vi "tcp_prepare_mode.vi"(0 "button_tcp_vna_mode":bool, 5 "button_tcp_s11_mode":bool, 7 "button_tcp_s21_mode":bool, 9 "button_tcp_smith_mode":bool, 12 "sweep_start":dbl, 13 "sweep_stop":dbl, 14 "sweep_points":dbl) -> (4 "mode":string, 6 "data_out":T1)   [LabVIEW 2025]
uses:
  2542fa05-10a6-4b30-b761-6670dfe4c8c8.vi
  647f14ae-cfaa-4bfc-9393-0c1ebd99a498.vi
  f7317db9-9ae3-40bd-acdc-ae7c641fa7e1.vi
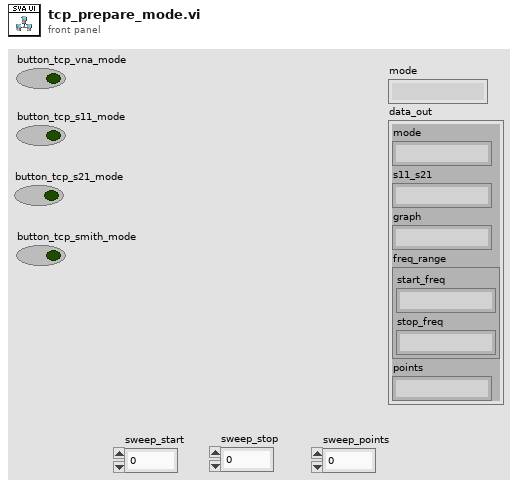
[diagram p1: front panel]
types:
  T1 = cluster{"mode":string, "s11_s21":string, "graph":string, "freq_range":cluster{"start_freq":string, "stop_freq":string}, "points":string}
  T2 = cluster{string, string, string, cluster{string, string}, string}
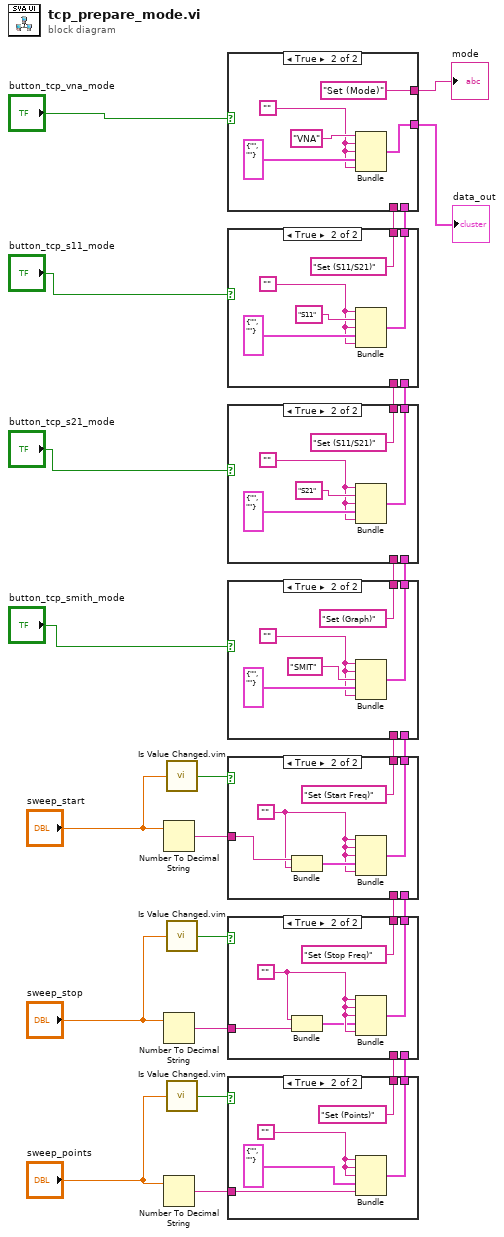
[diagram p0: block diagram]
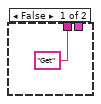
[diagram p2: hidden frame]
diagram:
  n1 = Number To Decimal String(number="sweep_start") -> (decimal integer string=w19:string)  [unwired: 1 in]
  n2 = Number To Decimal String(number="sweep_stop") -> (decimal integer string=w25:string)  [unwired: 1 in]
  n3 = Number To Decimal String(number="sweep_points") -> (decimal integer string=w3:string)  [unwired: 1 in]
  n4 = call "Is Value Changed.vim"("value"="sweep_start") -> ("changed or first call?"=w22:bool)
  n5 = call "Is Value Changed.vim"("value"="sweep_stop") -> ("changed or first call?"=w23:bool)
  n6 = call "Is Value Changed.vim"("value"="sweep_points") -> ("changed or first call?"=w5:bool)
  n7 = case shown="True" w5 {
    tunnel: ["Get" ("mode") "Set (Points)" ("mode")] -> w2
    tunnel: [_ w32] -> w1
    tunnel: w3 -> [_ w31]
    frame False {
    }
    frame True {
      w30 = ""
      n8 = Bundle(w30, w30, w30, cluster{string, string} {"", ""}, w31) -> (w32:T2)  [unwired: 1 in]
    }
  }
  n9 = case shown="True" w23 {
    tunnel: [w35 "Set (Stop Freq)" ("mode")] -> w26
    tunnel: [w34 w39] -> w27
    tunnel: w25 -> [_ w37]
    tunnel: w2 -> [w35 _]
    tunnel: w1 -> [w34 _]
    frame False {
    }
    frame True {
      w38 = ""
      n10 = Bundle(w38, w37) -> (w36:cluster{string, string})  [unwired: 1 in]
      n11 = Bundle(w38, w38, w38, w36, w38) -> (w39:T2)  [unwired: 1 in]
    }
  }
  n12 = case shown="True" w22 {
    tunnel: [w42 "Set (Start Freq)" ("mode")] -> w20
    tunnel: [w41 w46] -> w21
    tunnel: w19 -> [_ w45]
    tunnel: w26 -> [w42 _]
    tunnel: w27 -> [w41 _]
    frame False {
    }
    frame True {
      w43 = ""
      n13 = Bundle(w45, w43) -> (w44:cluster{string, string})  [unwired: 1 in]
      n14 = Bundle(w43, w43, w43, w44, w43) -> (w46:T2)  [unwired: 1 in]
    }
  }
  n15 = case shown="True" "button_tcp_smith_mode" {
    tunnel: [w49 "Set (Graph)" ("mode")] -> w12
    tunnel: [w48 w53] -> w13
    tunnel: w20 -> [w49 _]
    tunnel: w21 -> [w48 _]
    frame False {
    }
    frame True {
      w50 = ""
      n16 = Bundle(w50, w50, "SMIT", cluster{string, string} {"", ""}, w50) -> (w53:T2)  [unwired: 1 in]
    }
  }
  n17 = case shown="True" "button_tcp_s21_mode" {
    tunnel: [w56 "Set (S11/S21)" ("mode")] -> w10
    tunnel: [w55 w60] -> w11
    tunnel: w12 -> [w56 _]
    tunnel: w13 -> [w55 _]
    frame False {
    }
    frame True {
      w57 = ""
      n18 = Bundle(w57, "S21", w57, cluster{string, string} {"", ""}, w57) -> (w60:T2)  [unwired: 1 in]
    }
  }
  n19 = case shown="True" "button_tcp_s11_mode" {
    tunnel: [w63 "Set (S11/S21)" ("mode")] -> w8
    tunnel: [w62 w67] -> w9
    tunnel: w10 -> [w63 _]
    tunnel: w11 -> [w62 _]
    frame False {
    }
    frame True {
      w64 = ""
      n20 = Bundle(w64, "S11", w64, cluster{string, string} {"", ""}, w64) -> (w67:T2)  [unwired: 1 in]
    }
  }
  n21 = case shown="True" "button_tcp_vna_mode" {
    tunnel: [w70 "Set (Mode)" ("mode")] -> w6
    tunnel: [w69 w74] -> w7
    tunnel: w8 -> [w70 _]
    tunnel: w9 -> [w69 _]
    frame False {
    }
    frame True {
      w71 = ""
      n22 = Bundle("VNA", w71, w71, cluster{string, string} {"", ""}, w71) -> (w74:T2)  [unwired: 1 in]
    }
  }
  "data_out" <- w7
  "mode" <- w6
